vi "ziExample-Module-Impedance.vi"() -> ()   [LabVIEW 2009]
doc: "Control a Zurich instrument device via the LabOne Labview API. \nRequirements: Zurich Instruments MFLI+IA/ MFIA\nThis example shows how to use retrieve impedance data and utilize the sweeper.\n\n© Zurich Instruments AG, www.zhinst.com"
uses:
  <instrlib>/Zurich Instruments LabOne/Public/Modules/ziTypeModSweeperImpedanceWave.ctl
  <instrlib>/Zurich Instruments LabOne/Public/Modules/ziTypeModEnum.ctl
  <instrlib>/Zurich Instruments LabOne/Public/Configure/ziSetValueDoubleArray.vi
  <instrlib>/Zurich Instruments LabOne/Public/Modules/ziModSetValueDoubleArray.vi
  <instrlib>/Zurich Instruments LabOne/Public/Modules/ziModSetValueBinaryArray.vi
  <instrlib>/Zurich Instruments LabOne/Public/Modules/ziModGetSweeperData.vi
  <instrlib>/Zurich Instruments LabOne/Public/Configure/ziSetValueDouble.vi
  <instrlib>/Zurich Instruments LabOne/Public/Data/ziGetEventImpSample.vi
  <instrlib>/Zurich Instruments LabOne/Zurich Instruments LabOne.lvlib
  <vilib>/gmath/NI_Gmath.lvlib
panel:
  out "?":dbl(graph)
  out "?":dbl(graph)
  in  "Sweep":bool
  in  "Step":dbl=100.0
  in  "stopfreq":dbl=100000.0 caption="Stop Freq"
  in  "startfreq":dbl=1000.0 caption="Start Freq"
  in  "triggerautorange":bool caption="trigger autorange"
  in  "rangecontrol":u16(ring)=1 caption="Range Control" items=["Manual", "Auto"]
  out "Flags":bool[][](array[boolean])
  out "ImpedanceSweeperData":T1 {"bandwidthMode" format="%f"; "flags" format="%f"; "sampleFormat" format="%f"; "sweepMode" format="%f"; "sampleCount" format="%f"; "timestamp" format="%f"}
  in  "stop":bool
  out "Param1":dbl
  out "Param0":dbl format="%#_6p"
  out "Error Out":errorcluster
  in  "Address":string="DEV"
  out "Selected Device":string
  in  "subscribepath":string="imps/0/sample" caption="Subscribe Path"
  out "Param1":cluster{"grid":dbl[], "r_avg":dbl[]}(graph)
  out "Param 0":cluster{"grid":dbl[], "r_avg":dbl[]}(graph)
  # "ziExample-IMPModul.vi\nRequirements: MFLI + IA / MFIA\nsee block diagram for VI description"
  # "Tested Devices:\n\n- MFLI"
  # "VALID_INTERNAL\nVALID_USER\nAUTORANGE_GATING\n\nOVERFLOW_VOLTAGE\nOVERFLOW_CURRENT\nUNDERFLOW_VOLTAGE\nUNDERFLOW_CURRENT\nFREQ_EXACT\nFREQ_INTERPOLATION\nFREQ_EXTRAPOLATION\n\nSUPPRESSION_PARAM0\nSUPPRESSION_PARAM1\nFREQLIMIT_RANGE_VOLTAGE\nFREQLIMIT_RANGE_Current\nSTRONGCOMPENSATION_PARAM0\nSTRONGCOMPENSATION_PARAM1\n\n\nBWC_BIT0\nBWC_BIT1\nBWC_BIT2\nBWC_BIT3\nOPEN_DETECTION"
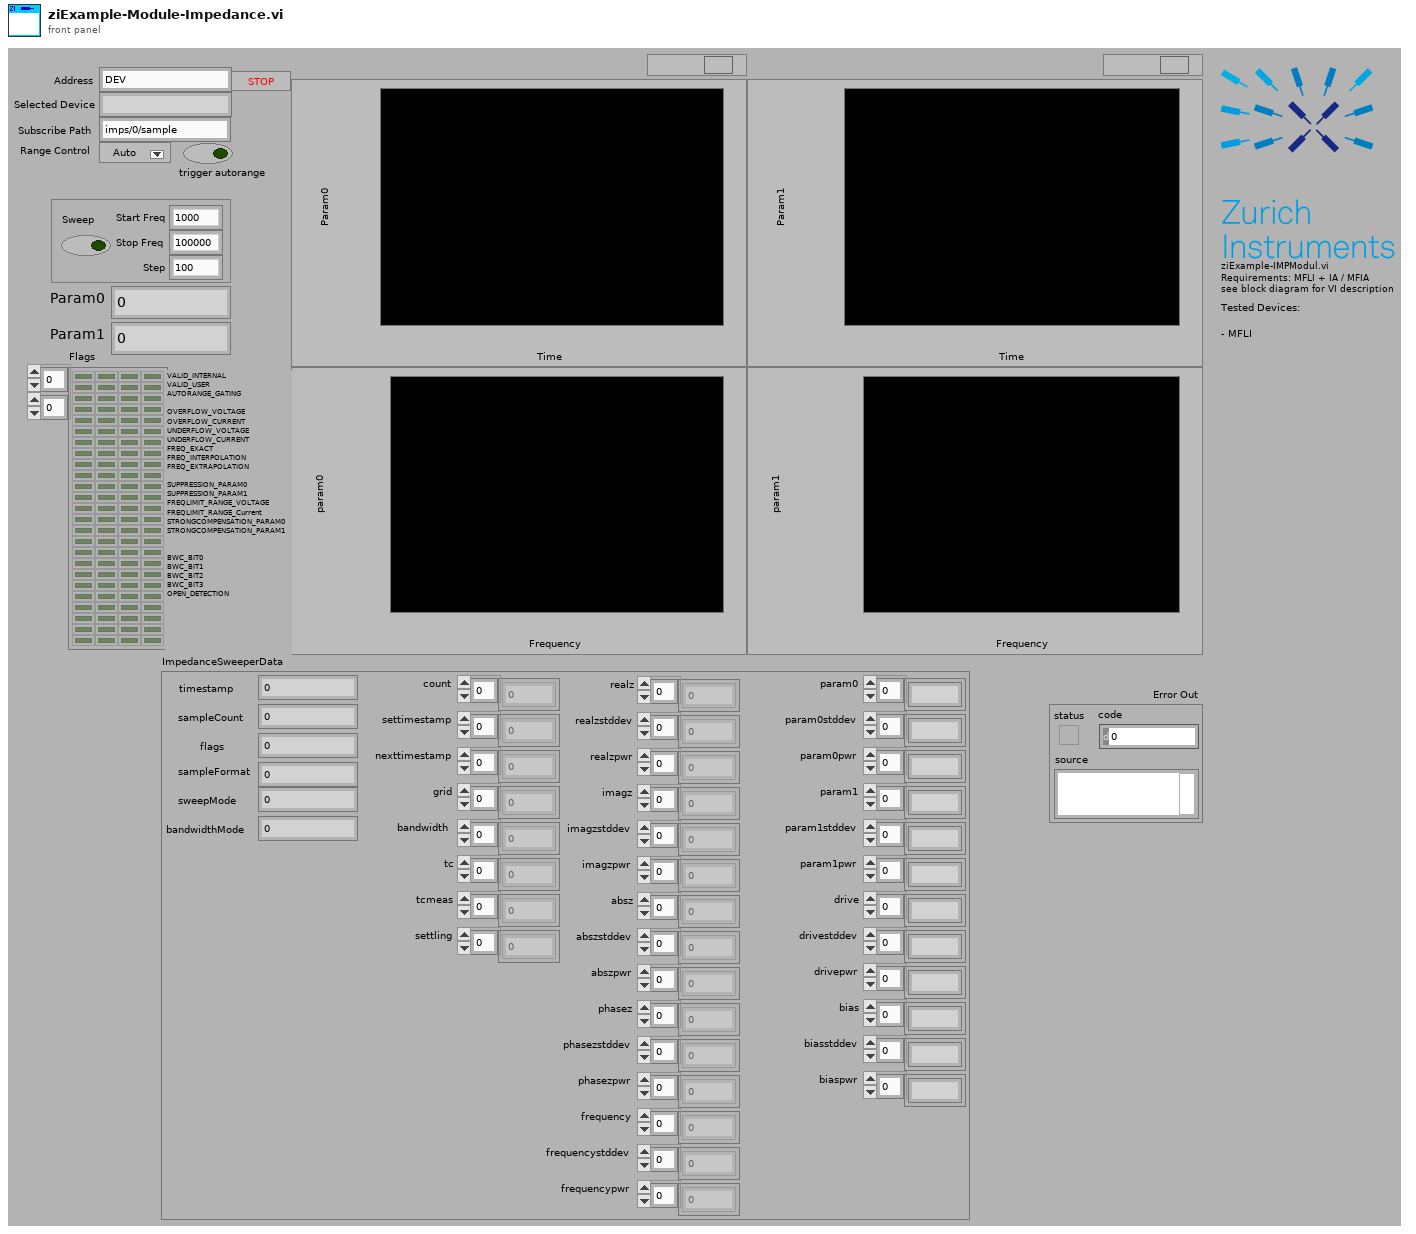
[diagram p1: front panel]
types:
  T1 = typedef "Zurich Instruments LabOne.lvlib/ziTypeModSweeperImpedanceWave.ctl" = cluster{"timestamp":u64, "sampleCount":u64, "flags":u8, "sampleFormat":u8, "sweepMode":u8, "bandwidthMode":u8, "count":u64[], "settimestamp":u64[], "nexttimestamp":u64[], "grid":dbl[], "bandwidth":dbl[], "tc":dbl[], "tcmeas":dbl[], "settling":dbl[], "realz":dbl[], "realzstddev":dbl[], "realzpwr":dbl[], "imagz":dbl[], "imagzstddev":dbl[], "imagzpwr":dbl[], "absz":dbl[], "abszstddev":dbl[], "abszpwr":dbl[], "phasez":dbl[], "phasezstddev":dbl[], "phasezpwr":dbl[], "frequency":dbl[], "frequencystddev":dbl[], "frequencypwr":dbl[], "param0":dbl[], "param0stddev":dbl[], "param0pwr":dbl[], "param1":dbl[], "param1stddev":dbl[], "param1pwr":dbl[], "drive":dbl[], "drivestddev":dbl[], "drivepwr":dbl[], "bias":dbl[], "biasstddev":dbl[], "biaspwr":dbl[]}
  T2 = typedef "Zurich Instruments LabOne.lvlib/ziTypeModEnum.ctl" = u16
  T3 = typedef "Zurich Instruments LabOne.lvlib/ziTypeHandle.ctl" = cluster{"handleValid":bool, "Conn":u64, "Path Prefix":string, "Handle":u64, "Connected":bool, "Clockbase(s)":dbl}
  T4 = typedef "Zurich Instruments LabOne.lvlib/ziTypeModHandle.ctl" = cluster{"handleValid":bool, "Conn":u64, "ModHandle":u64, "moduleID":string, "Path Prefix":string}
  T5 = typedef "Zurich Instruments LabOne.lvlib/ziTypeModResults.ctl" = cluster{"PathArray":string[], "ValueType":T6, "NoOfResults":u64, "ziGenericHeader":T7[]}
  T6 = typedef "Zurich Instruments LabOne.lvlib/ziTypePollType.ctl" = enum16{"NONE", "DOUBLE_DATA", "INTEGER_DATA", "DEMOD_SAMPLE", "SCOPE_WAVE_HF2", "AUXIN_SAMPLE", "DIO_SAMPLE", "BYTE_ARRAY", "PWA_WAVE", "9", "10", "11", "12", "13", "14", "15", "TREE_CHANGE_DEPRI", "17", "ERROR", "19", "20", "21", "22", "23", "24", "25", "26", "27", "28", "29", "30", "31", "DOUBLE_DATA_TS", "INTEGER_DATA_TS", "34", "SCOPE_WAVE", "SCOPE_WAVE_EX", "37", "BYTE_ARRAY_TS", "39", "40", "41", "42", "43", "44", "45", "CNT_DATA", "47", "TREE_CHANGE", "49", "50", "51", "52", "53", "54", "55", "56", "57", "58", "59", "60", "61", "62", "63", "SWEEPER_DATA", "SPECTRUM_DATA", "ADVISOR_DATA", "VECTOR_DATA", "IMP_DATA"}
  T7 = typedef "Zurich Instruments LabOne.lvlib/ziTypeModGenericHeader.ctl" = cluster{"HeaderType":enum8{"HEADER_TYPE_NONE", "HEADER_TYPE_SWTRIGGER", "HEADER_TYPE_SWEEPER"}, "SampleFormat":u8, "SystemTime":timestamp, "CreatedTimeStamp":u64, "ChangedTimeStamp":u64, "Flags":u32, "ChunkSizeBytes":u64, "Name":string, "Status":u32, "GroupIndex":u32, "Color":u32, "ActiveRow":u32, "TriggerNumber":u64, "GridRows":u32, "GridCols":u32, "GridMode":u32, "GridOperation":u32, "GridDirection":u32, "GridRepetitions":u32, "GridColDelta":dbl, "GridColOffset":dbl, "GridRowDelta":dbl, "GridRowOffset":dbl, "Bandwidth":dbl, "Center":dbl, "Nenbw":dbl}
  T8 = typedef "Zurich Instruments LabOne.lvlib/ziTypeImpedanceSample.ctl" = cluster{"Timestamps (ticks)":u64[], "Z (Ohm)":cdb[], "Freq (Hz)":dbl[], "Osc Phase (deg)":dbl[], "Flags":u32[], "Trigger":u32[], "Param0":dbl[], "Param1":dbl[], "Drive":dbl[], "Bias":dbl[]}
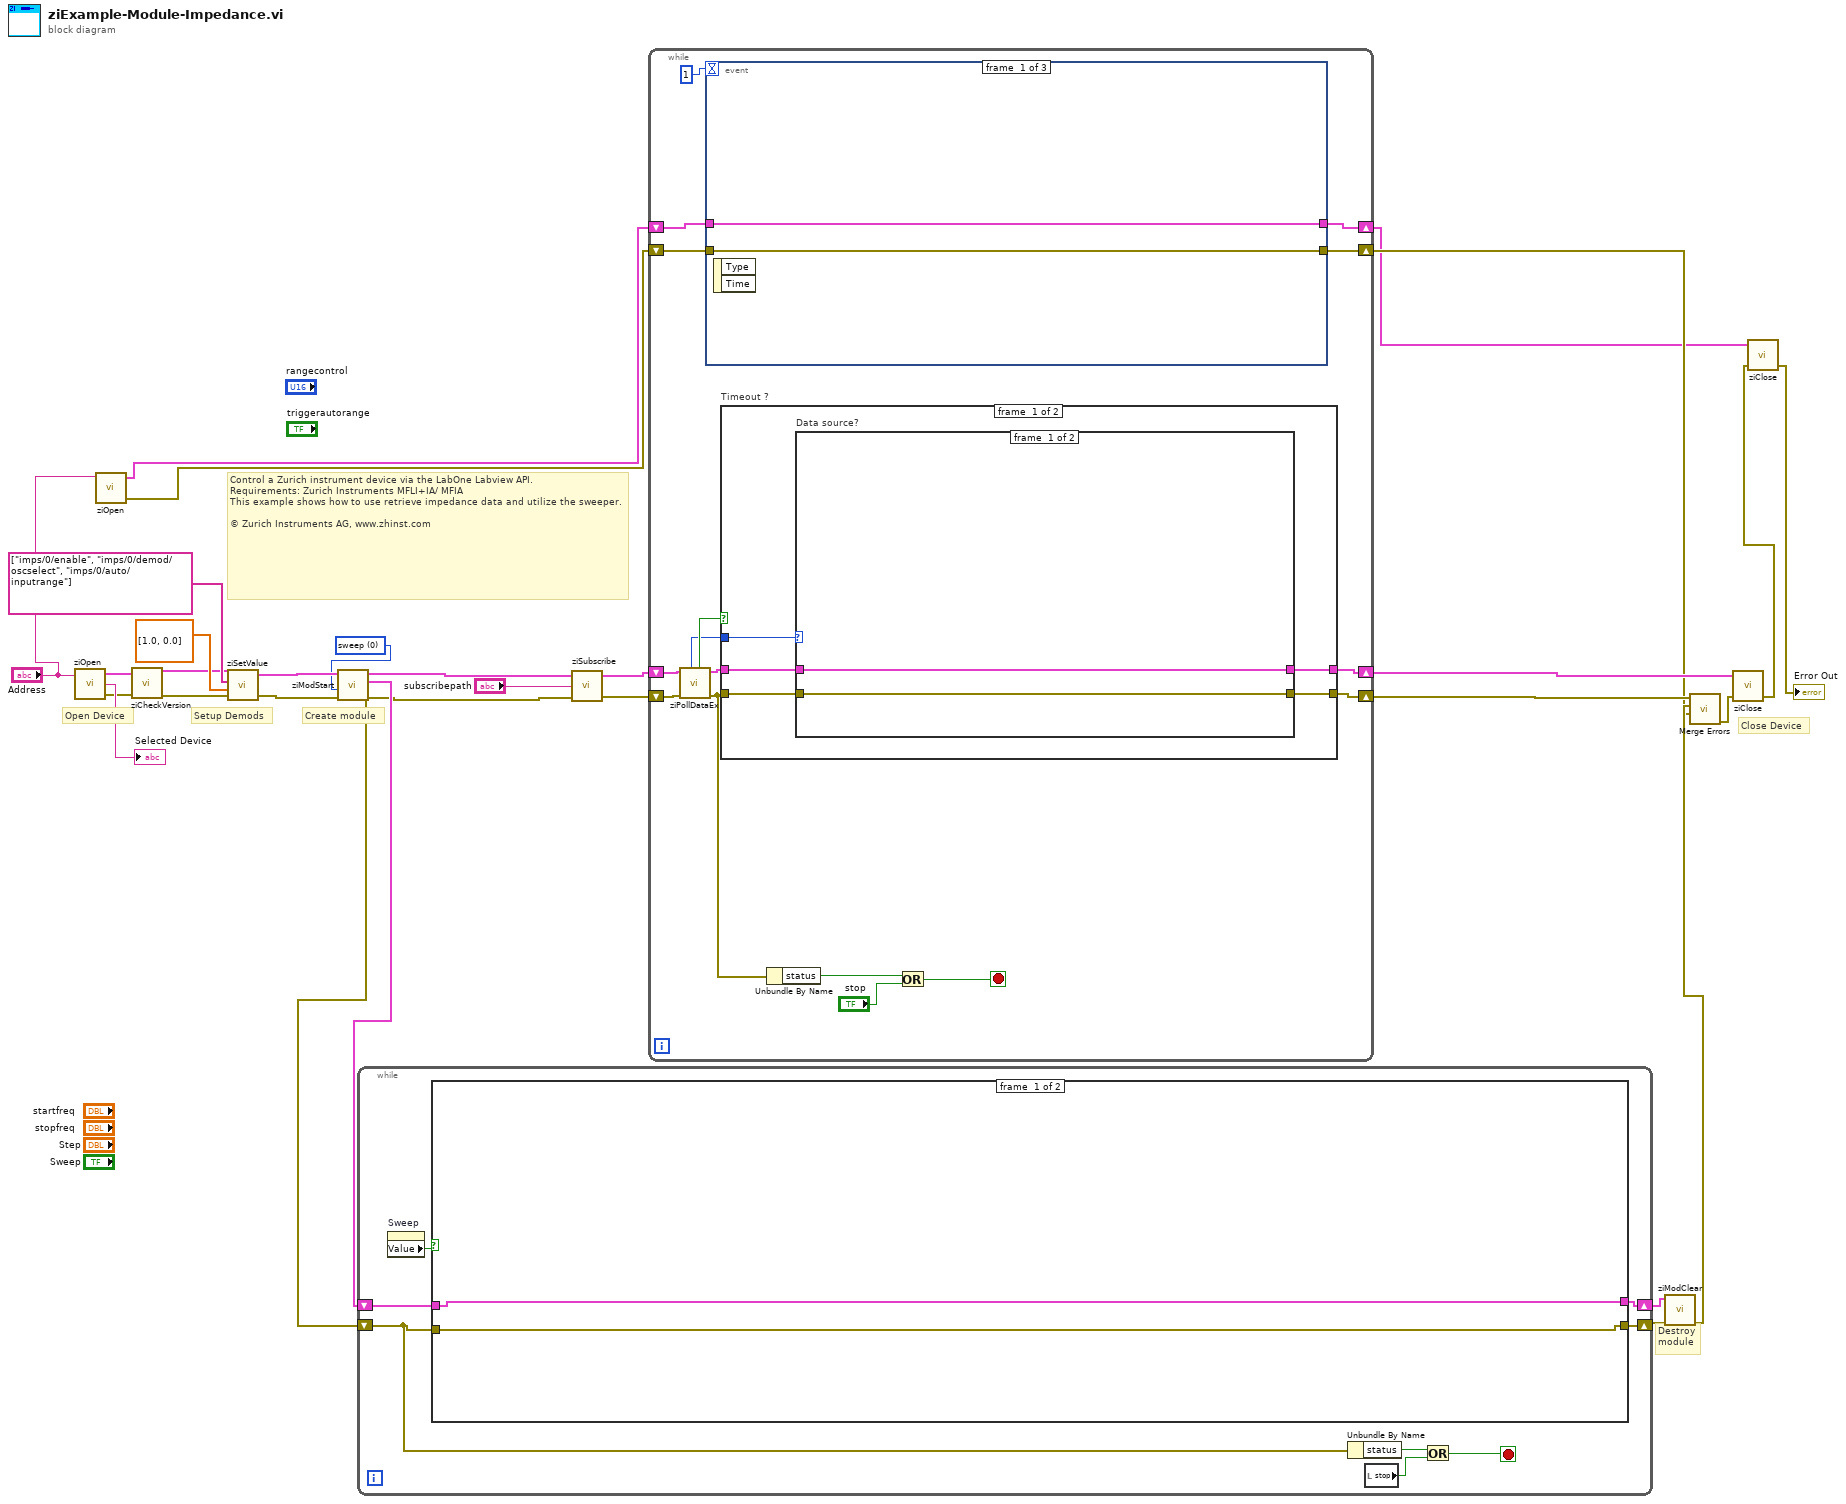
[diagram p0: block diagram]
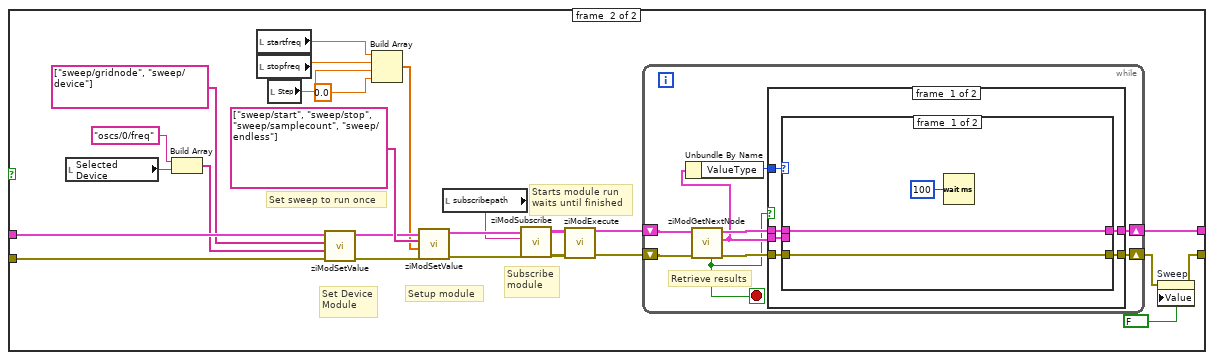
[diagram p2: hidden frame]
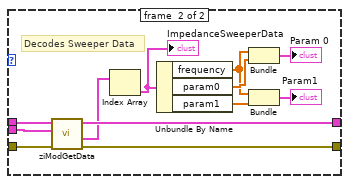
[diagram p3: hidden frame]
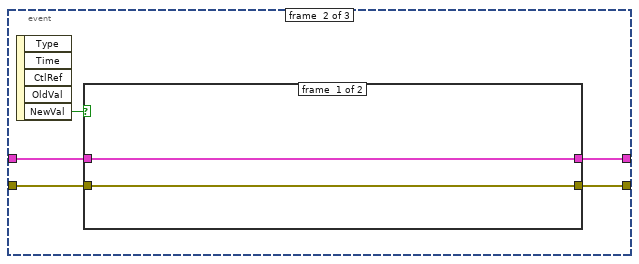
[diagram p5: hidden frame]
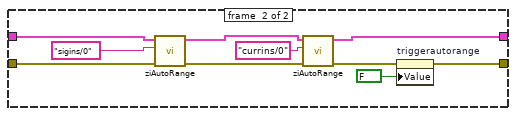
[diagram p6: hidden frame]
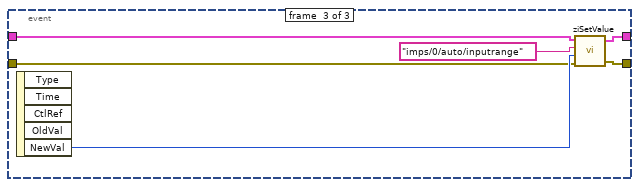
[diagram p7: hidden frame]
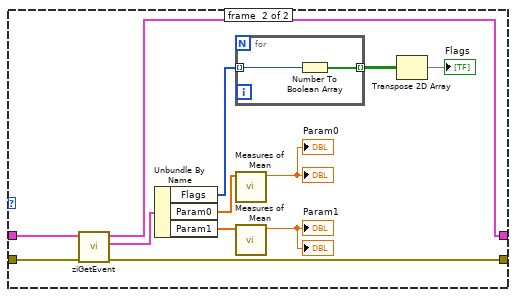
[diagram p8: hidden frame]
diagram:
  w8 = T2 0 items=["sweep", "scopeModule", "dataAcquisitionModule", "pidAdvisor", "awgModule", "impedanceModule", "multiDeviceSyncModule", "zoomFFT", "trigger", "deviceSettings", "record"] ("module Id")
  # "Destroy\nmodule"
  # "Control a Zurich instrument device via the LabOne Labview API. \nRequirements: Zurich Instruments MFLI+IA/ MFIA\nThis example shows how to use retrieve impedance data and utilize the sweeper.\n\n© Zurich Instruments AG, www.zhinst.com"
  # "Setup Demods"
  # "Create module"
  # "Close Device"
  # "Open Device"
  n1 = call <instrlib>:"ziOpen.vi"("Address"="Address") -> ("Error Out"=w11:errorcluster, "Selected Device"=→"Selected Device":string, "HandleOut"=w12:T3)  [unwired: 1 in, 2 out]
  n2 = call <instrlib>:"ziOpen.vi"("Address"="Address") -> ("Error Out"=w5:errorcluster, "HandleOut"=w6:T3)  [unwired: 1 in, 3 out]
  n3 = call <instrlib>:"ziCheckVersion.vi"("Handle In"=w12, "Error In"=w11) -> ("Handle Out"=w9:T3, "Error Out"=w10:errorcluster)  [unwired: 11 in, 1 out]
  n4 = call-poly <instrlib>:"ziSetValue.vi"("Error In"=w10, "Values"=dbl[] [1.0, 0.0], "Paths"=string[] ["imps/0/enable", "imps/0/demod/oscselect", "imps/0/auto/inputrange"], "Handle In"=w9) -> ("Error Out"=w14:errorcluster, "Handle Out"=w15:T3)  [unwired: 1 in]
  n5 = call <instrlib>:"ziModStart.vi"("Error In"=w14, "module Id"=w8, "Handle In"=w15) -> ("Error Out"=w20:errorcluster, "ModHandle Out"=w28:T4, "Handle Out"=w23:T3)  [unwired: 6 in]
  n6 = while {
    shift-right: [w35] -> w25
    shift-left: w28 -> [w37]
    shift-right: [w36] -> w26
    shift-left: w20 -> [w33]
    stop <- w30 stop-if-true
    n7 = property on="Sweep" class="Bool (strict)"() -> ("Value"=w34:bool)  [unwired: 2 in, 2 out]
    n8 = case shown="False" w34 {
      tunnel: w37 -> [w39 w64]
      tunnel: [w38 w63] -> w36
      tunnel: [w39 w62] -> w35
      tunnel: w33 -> [w38 w61]
      frame #0 {
      }
      frame #1 {
        # "Set Device\nModule"
        # "Starts module run\nwaits until finished"
        # "Set sweep to run once"
        # "Subscribe\nmodule"
        # "Setup module"
        n9 = local read "Selected Device"() -> (w48:string)
        n10 = Build Array("oscs/0/freq", w48) -> (w46:string[])
        n11 = local read "startfreq"() -> (w42:dbl)
        n12 = local read "stopfreq"() -> (w41:dbl)
        n13 = local read "Step"() -> (w40:dbl)
        n14 = call-poly <instrlib>:"ziModSetValue.vi"("Error In"=w61, "Values"=w46, "Paths"=string[] ["sweep/gridnode", "sweep/device"], "ModHandle In"=w64) -> ("Error Out"=w54:errorcluster, "ModHandle Out"=w57:T4)  [unwired: 6 in]
        n15 = Build Array(w42, w41, w40, 0.0 ("Value")) -> (w49:dbl[])
        n16 = call-poly <instrlib>:"ziModSetValue.vi"("Error In"=w54, "Values"=w49, "Paths"=string[] ["sweep/start", "sweep/stop", "sweep/samplecount", "sweep/endless"], "ModHandle In"=w57) -> ("Error Out"=w55:errorcluster, "ModHandle Out"=w56:T4)  [unwired: 6 in]
        n17 = local read "subscribepath"() -> (w53:string)
        n18 = call <instrlib>:"ziModSubscribe.vi"("Error In"=w55, "Path"=w53, "ModHandle In"=w56) -> ("Error Out"=w50:errorcluster, "ModHandle Out"=w51:T4)  [unwired: 6 in]
        n19 = call <instrlib>:"ziModExecute.vi"("Error In"=w50, "ziModHandle In"=w51) -> ("Error Out"=w59:errorcluster, "ziModHandle Out"=w60:T4)  [unwired: 6 in, 1 out]
        n20 = while {
          shift-right: [w70] -> w62
          shift-left: w60 -> [w72]
          shift-right: [w69] -> w44
          shift-left: w59 -> [w73]
          stop <- w65 stop-if-true
          # "Retrieve results"
          n21 = call <instrlib>:"ziModGetNextNode.vi"("Error In"=w73, "ModHandle In"=w72) -> ("Error Out"=w66:errorcluster, "ModResults"=w68:T5, "ModHandle Out"=w71:T4, "NoData"=w65:bool)  [unwired: 6 in]
          n22 = Unbundle By Name(w68) -> ("ValueType"=w67:T6)
          n23 = case shown="False" w65 {
            tunnel: w71 -> [w79 w95]
            tunnel: [w78 w95] -> w70
            tunnel: [w77 w96] -> w69
            tunnel: w66 -> [w76 w96]
            tunnel: w68 -> [w75 _]
            tunnel: w67 -> [w74 _]
            frame #0 {
              n24 = case shown="\"SWEEPER_DATA\"" w74 {
                tunnel: w79 -> [w82 w93]
                tunnel: w75 -> [_ w94]
                tunnel: w76 -> [w81 w92]
                tunnel: [w81 w91] -> w77
                tunnel: [w82 w90] -> w78
                frame #0 {
                  n25 = Wait (ms)(milliseconds to wait=u32 100) -> ()  [unwired: 1 out]
                }
                frame #1 {
                  # "Decodes Sweeper Data"
                  n26 = call-poly <instrlib>:"ziModGetData.vi"("Error In"=w92, "ModResults"=w94, "ModHandle In"=w93) -> ("Error Out"=w91:errorcluster, "SweeperImpedanceWaveArray"=w84:T1[], "ModHandle Out"=w90:T4)  [unwired: 4 in, 2 out]
                  n27 = Index Array(array=w84) -> (element=w83:T1)  [unwired: 1 in]
                  "ImpedanceSweeperData" <- w83
                  n28 = Unbundle By Name(w83) -> ("frequency"=w85:dbl[], "param0"=w89:dbl[], "param1"=w86:dbl[])
                  n29 = Bundle("frequency"=w85, "param0"=w89) -> (→"Param 0":cluster{"frequency":dbl[], "param0":dbl[]})  [unwired: 1 in]
                  n30 = Bundle("frequency"=w85, "param1"=w86) -> (→"Param1":cluster{"frequency":dbl[], "param1":dbl[]})  [unwired: 1 in]
                }
              }
            }
            frame #1 {
            }
          }
        }
        n31 = property on="Sweep" class="Bool (strict)"(error in=w44, "Value"=FALSE ("Sweep")) -> (error out=w63:errorcluster)  [unwired: 1 in, 1 out]
      }
    }
    n32 = Unbundle By Name(w33) -> ("status"=w31:bool)
    n33 = local read "stop"() -> (w32:bool)
    n34 = Or(x=w31, y=w32) -> (x .or. y?=w30:bool)
  }
  n35 = call <instrlib>:"ziSubscribe.vi"("error in"=w20, "Path ()"="subscribepath", "Handle In"=w23) -> ("error out"=w21:errorcluster, "Handle Out"=w22:T3)  [unwired: 1 in]
  n36 = while {
    shift-right: [w109] -> w18
    shift-left: w21 -> [w101]
    shift-right: [w110] -> w24
    shift-left: w22 -> [w102]
    shift-right: [w98] -> w2
    shift-left: w6 -> [w100]
    shift-right: [w97] -> w4
    shift-left: w5 -> [w99]
    stop <- w103 stop-if-true
    n37 = call <instrlib>:"ziPollDataEx.vi"("error in"=w101, "Handle In"=w102) -> ("error out"=w106:errorcluster, "Handle Out"=w111:T3, "Timed Out"=w112:bool, "ziValueType"=w108:T6)  [unwired: 2 in, 4 out]
    n38 = event shown="[1] \"triggerautorange\": Value Change" {
      selector: _ -> [_ _ _]
      dyn-events: _ -> [_ _ _]
      timeout: 1 -> [_ _ _]
      tunnel: w100 -> [w114 w118 w135]
      tunnel: w99 -> [w113 w119 w134]
      tunnel: [w114 w117 w133] -> w98
      tunnel: [w113 w116 w132] -> w97
      event #0 {
        n39 = event-data() -> ()  [unwired: 1 in, 2 out]
      }
      event #1 {
        n40 = event-data() -> ("NewVal"=w115:bool)  [unwired: 1 in, 4 out]
        n41 = case shown="True" w115 {
          tunnel: w119 -> [w120 w128]
          tunnel: [w120 w122] -> w116
          tunnel: [w121 w129] -> w117
          tunnel: w118 -> [w121 w131]
          frame #0 {
          }
          frame #1 {
            n42 = call <instrlib>:"ziAutoRange.vi"("Error in"=w128, "Path"="sigins/0", "Handle in"=w131) -> ("Error out"=w127:errorcluster, "Handle out"=w130:T3)  [unwired: 6 in, 1 out]
            n43 = call <instrlib>:"ziAutoRange.vi"("Error in"=w127, "Path"="currins/0", "Handle in"=w130) -> ("Error out"=w123:errorcluster, "Handle out"=w129:T3)  [unwired: 6 in, 1 out]
            n44 = property on="triggerautorange" class="Bool (strict)"(error in=w123, "Value"=FALSE) -> (error out=w122:errorcluster)  [unwired: 1 in, 1 out]
          }
        }
      }
      event #2 {
        n45 = event-data() -> ("NewVal"=w136:u16)  [unwired: 1 in, 4 out]
        n46 = call-poly <instrlib>:"ziSetValue.vi"("Error In"=w134, "Value"=w136, "Path"="imps/0/auto/inputrange", "Handle In"=w135) -> ("Error Out"=w132:errorcluster, "Handle Out"=w133:T3)  [unwired: 1 in]
      }
    }
    n47 = case "Timeout ?" shown="False" w112 {
      tunnel: w111 -> [w142 w160]
      tunnel: [w141 w160] -> w110
      tunnel: w106 -> [w140 w159]
      tunnel: [w139 w159] -> w109
      tunnel: w108 -> [w138 _]
      frame #0 {
        n48 = case "Data source?" shown="\"IMP_DATA\"" w138 {
          tunnel: w142 -> [w144 w156]
          tunnel: [w144 w152] -> w141
          tunnel: w140 -> [w143 w154]
          tunnel: [w143 w153] -> w139
          frame #0 {
          }
          frame #1 {
            n49 = call-poly <instrlib>:"ziGetEvent.vi"("Error In"=w154, "Handle In"=w156) -> ("Error Out"=w153:errorcluster, "Imp Sample Out"=w155:T8, "Handle Out"=w152:T3)  [unwired: 7 in]
            n50 = Unbundle By Name(w155) -> ("Flags"=w151:u32[], "Param0"=w148:dbl[], "Param1"=w147:dbl[])
            n51 = for {
              tunnel: w151 -> [w158] mode=indexing
              tunnel: [w157] -> w150 mode=indexing
              n52 = Number To Boolean Array(number=w158) -> (Boolean array=w157:bool[])
            }
            n53 = call <vilib>:"Measures of Mean.vi"("x array"=w148) -> ("mean value"=→"Param0" →"?":dbl)  [unwired: 9 in, 1 out]
            n54 = call <vilib>:"Measures of Mean.vi"("x array"=w147) -> ("mean value"=→"Param1" →"?":dbl)  [unwired: 9 in, 1 out]
            n55 = Transpose 2D Array(2D array=w150) -> (transposed array=→"Flags":bool[][])
          }
        }
      }
      frame #1 {
        # "Timeout, no action."
      }
    }
    n56 = Unbundle By Name(w106) -> ("status"=w104:bool)
    n57 = Or(x=w104, y="stop") -> (x .or. y?=w103:bool)
  }
  n58 = call <instrlib>:"ziModClear.vi"("Error In"=w26, "ziModHandle In"=w25) -> ("Error Out"=w19:errorcluster)  [unwired: 7 in, 1 out]
  n59 = call <vilib>:"Merge Errors.vi"("error in 3 (no error)"=w4, "error in 2 (no error)"=w19, "error in 1 (no error)"=w18) -> ("error out"=w17:errorcluster)  [unwired: 4 in]
  n60 = call <instrlib>:"ziClose.vi"("Error In"=w17, "Handle In"=w24) -> ("Error Out"=w3:errorcluster)  [unwired: 2 in, 1 out]
  n61 = call <instrlib>:"ziClose.vi"("Error In"=w3, "Handle In"=w2) -> ("Error Out"=→"Error Out":errorcluster)  [unwired: 2 in, 1 out]
